vi "Write queue size.vi"(8 "error in (no error)":errorcluster, 10 "queue size":u16=25, 11 "TDMS datalogger configuration in":refnum<class "TDMS datalogger configuration.lvclass">) -> (0 "error out":errorcluster, 3 "TDMS datalogger configuration out":refnum<class "TDMS datalogger configuration.lvclass">)   [LabVIEW 2013, in "TDMS datalogger configuration.lvclass"]
uses:
  TDMS datalogger configuration.lvclass
  TDMS datalogger configuration.lvclass/TDMS datalogger configuration.ctl
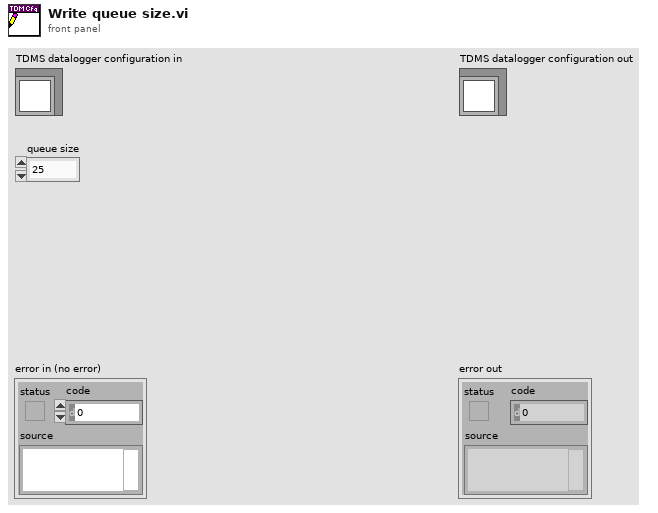
[diagram p1: front panel]
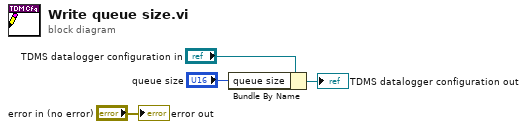
[diagram p0: block diagram]
diagram:
  n1 = Bundle By Name(cluster="TDMS datalogger configuration in", "queue size"="queue size") -> (→"TDMS datalogger configuration out":refnum<class "TDMS datalogger configuration.lvclass">)
  "error out" <- "error in (no error)"
